vi "SetUpLeCroy.vi"(6 "Therapy (T)":bool, 7 "Therapy VISA session":refnum<visa-resource-name>, 8 "Ann Array Params":T2={"Synth Foc?"=FALSE, "Focal Zones"=41, "Switch T/R"=0, "Trans Geometry (mm)"={"Transducer"=0, "Geo Focus"=12.0, "a (radius)"=3.0, "# of rings"=5, "kerf space "=0.1, "Center Freq"=12.0}, "Sub Ap Excite?"=FALSE, "Full Array Scan?"=FALSE, "Xmt/Rcv"={"XMIT"=[TRUE, TRUE, TRUE, TRUE, TRUE], "RCV"=[TRUE, TRUE, TRUE, TRUE, TRUE]}, "PulseSpacing (us)"=0.0, "Xmit Ring"=0, "XMIT CHS"=0, "RCV CHS"=0, "GPU?"=FALSE, "Save TIFF?"=FALSE, "downfactor"=1, "RCV 1CH"=0} {"RCV 1CH" items=["All", "1", "2", "3", "4", "5"]; "Trans Geometry (mm)"."Transducer" items=["6D 12R 40 MHz"=0, "10D 31R 20 MHz"=1, "10D 23R 20 MHz"=2, "6D 23R 40 MHz"=3, "4.5D 10.7R 40 MHz"=4, "9D 23.5R 20 MHz"=5, "9D 25.8R 20MHz"=6, "Enter"=99]; "Switch T/R" min=1 max=5 step=1}, 10 "Motion Settings In":T6={"No Motion?"=FALSE, "Motion System"=enum."NI 735x", "Motion Bd ID"=1, "Motion Profile"="SMAC1", "# Axis"=1, "Reverse Z axis?"=TRUE, "SMAC Axis"=0, "scan pair"=enum."y-(x) scan", "RT fps"=6.0, "Steps per mm"=[1000, 1000, 1000, 1000], "Motor Parameters"={"velocity ct/s"=[10000.0, 10000.0, 10000.0, 50000.0], "accel ct/s^2"=[50000.0, 50000.0, 50000.0, 200000.0]}, "One Way Scan"=FALSE, "Reverse One Way Scan"=FALSE, "Global Position (mm)"=[], "Plane"=0, "Distance between\nscan lines (um)"=0.0, "Distance between\nscan planes (um)"=0.0, "number of scan planes"=1, "Total steps in line"=0, "Xtra plane\ndistance  (um)"=100, "Xtra planes "=1, "Add Axis"=FALSE, "overshoot cts"=200, "BKPT Shift"=0, "Scan Start Time (ms)"=0, "ESP VISA"="GPIB::1::INSTR", "3rd Axis"=1, "GL Ref Out"=refnum, "Galil Address"=""} {"3rd Axis" items=["x", "y", "z", "w"]; "Xtra planes" min=1; "Xtra plane\ndistance  (um)" min=0; "Distance between\nscan planes (um)" format="%.2f"; "Distance between\nscan lines (um)" format="%.2f"; "SMAC Axis" items=["None"=0, "Axis 1"=1, "Axis 2"=2, "Axis 3"=3, "Axis 4"=4, "Axis 5"=5, "Axis 6"=6, "Axis 7"=7, "Axis 8"=8, "Vector Space 1"=17, "Vector Space 2"=18, "Vector Space 3"=19, "Vector Space 4"=20]; "Motion Bd ID" min=1 max=32 step=1}, 11 "Digitizer Settings":T10={"Digitizer delay (us) "=0.0, "rf points per line"=2048, "lines per plane"=128, "Samp Rate (Hz)"=100000000.0, "Additional dig delay (us)"=0.0, "Voltage Scale"=0.4, "Pre-Looks"=0, "Offset delay (us)"=0.0, "bits A/D"=8, "Avg Num"=1, "DigTimeOut"=5.0, "Rel Dig Delay"=0.0, "Dig Ch"=0, "LeCroyCluster"={"LeCroy Channels"=[TRUE, FALSE, FALSE, FALSE], "LC read pt offset"=0.0, "Sweep Avg"=FALSE}, "Main Digitizer"=enum."NI Digitizer", "Dig Config"=enum."Single channel", "Digitizer ID Cluster"={"Acqiris/Alazar/SP ID"=[], "NI Instr Handles"=[], "LeCroy VISA"="", "GaGe Handle"={"Handle"=0, "Sample size"=0, "Resolution"=0, "Offset"=0, "Channels"=0, "Boards"=0}, "ATS Ref"="ATS9350", "Acqiris Address"=["PCI::INSTR0"], "ADQRef"=refnum, "adq_cu_ptr"=refnum}, "Trigger Settings"={"Trig Source"=1, "Trig Coupling"=0, "Trig Slope"=0, "Level (mV)"=1500.0}, "Bulk Acq"=FALSE, "Bulk Start Indexes"=[], "Data Ref RF"=refnum, "NI ID/Channel"=[], "Total Dig CH"=1, "Xtra Ann Trig delay (us)"=10.0, "Fix Z Delay?"=FALSE, "One Way Transmission?"=FALSE, "Data Ref Log"=refnum} {"Trigger Settings"."Trig Slope" items=["Positive", "Negative"]; "Trigger Settings"."Level (mV)" format="%.2f"; "Trigger Settings"."Trig Coupling" items=["DC 1 MOhm", "AC 1 MOhm", "DC 50 Ohm", "AC 50 Ohm"]; "Trigger Settings"."Trig Source" items=["Chan 1", "External"]; "Rel Dig Delay" format="%.2f"; "DigTimeOut" format="%.2f"; "Avg Num" min=1; "Offset delay (us)" format="%.2f"; "Additional dig delay (us)" format="%.2f"; "Digitizer delay (us)" format="%.2f"}) -> (0 "Waveform Graph":cluster{i32, dbl, dbl[]}(graph), 1 "Equivalent RT delay\ndistance (mm)":dbl=1.5 format="%.4f", 2 "Motion Settings Out":T6={"No Motion?"=FALSE, "Motion System"=enum."NI 735x", "Motion Bd ID"=1, "Motion Profile"="SMAC1", "# Axis"=1, "Reverse Z axis?"=TRUE, "SMAC Axis"=0, "scan pair"=enum."y-(x) scan", "RT fps"=6.0, "Steps per mm"=[1000, 1000, 1000, 1000], "Motor Parameters"={"velocity ct/s"=[10000.0, 10000.0, 10000.0, 50000.0], "accel ct/s^2"=[50000.0, 50000.0, 50000.0, 200000.0]}, "One Way Scan"=FALSE, "Reverse One Way Scan"=FALSE, "Global Position (mm)"=[], "Plane"=0, "Distance between\nscan lines (um)"=0.0, "Distance between\nscan planes (um)"=0.0, "number of scan planes"=1, "Total steps in line"=0, "Xtra plane\ndistance  (um)"=100, "Xtra planes "=1, "Add Axis"=FALSE, "overshoot cts"=200, "BKPT Shift"=0, "Scan Start Time (ms)"=0, "ESP VISA"="GPIB::1::INSTR", "3rd Axis"=1, "GL Ref Out"=refnum, "Galil Address"=""} {"3rd Axis" items=["x", "y", "z", "w"]; "Xtra planes" min=1; "Xtra plane\ndistance  (um)" min=0; "Distance between\nscan planes (um)" format="%.2f"; "Distance between\nscan lines (um)" format="%.2f"; "SMAC Axis" items=["None"=0, "Axis 1"=1, "Axis 2"=2, "Axis 3"=3, "Axis 4"=4, "Axis 5"=5, "Axis 6"=6, "Axis 7"=7, "Axis 8"=8, "Vector Space 1"=17, "Vector Space 2"=18, "Vector Space 3"=19, "Vector Space 4"=20]; "Motion Bd ID" min=1 max=32 step=1}, 3 "Ann Array Params out":T2={"Synth Foc?"=FALSE, "Focal Zones"=41, "Switch T/R"=0, "Trans Geometry (mm)"={"Transducer"=0, "Geo Focus"=12.0, "a (radius)"=3.0, "# of rings"=5, "kerf space "=0.1, "Center Freq"=12.0}, "Sub Ap Excite?"=FALSE, "Full Array Scan?"=FALSE, "Xmt/Rcv"={"XMIT"=[TRUE, TRUE, TRUE, TRUE, TRUE], "RCV"=[TRUE, TRUE, TRUE, TRUE, TRUE]}, "PulseSpacing (us)"=0.0, "Xmit Ring"=0, "XMIT CHS"=0, "RCV CHS"=0, "GPU?"=FALSE, "Save TIFF?"=FALSE, "downfactor"=1, "RCV 1CH"=0} {"RCV 1CH" items=["All", "1", "2", "3", "4", "5"]; "Trans Geometry (mm)"."Transducer" items=["6D 12R 40 MHz"=0, "10D 31R 20 MHz"=1, "10D 23R 20 MHz"=2, "6D 23R 40 MHz"=3, "4.5D 10.7R 40 MHz"=4, "9D 23.5R 20 MHz"=5, "9D 25.8R 20MHz"=6, "Enter"=99]; "Switch T/R" min=1 max=5 step=1}, 4 "Digitizer Settings Out":T10={"Digitizer delay (us) "=0.0, "rf points per line"=2048, "lines per plane"=128, "Samp Rate (Hz)"=100000000.0, "Additional dig delay (us)"=0.0, "Voltage Scale"=0.4, "Pre-Looks"=0, "Offset delay (us)"=0.0, "bits A/D"=8, "Avg Num"=1, "DigTimeOut"=5.0, "Rel Dig Delay"=0.0, "Dig Ch"=0, "LeCroyCluster"={"LeCroy Channels"=[TRUE, FALSE, FALSE, FALSE], "LC read pt offset"=0.0, "Sweep Avg"=FALSE}, "Main Digitizer"=enum."NI Digitizer", "Dig Config"=enum."Single channel", "Digitizer ID Cluster"={"Acqiris/Alazar/SP ID"=[], "NI Instr Handles"=[], "LeCroy VISA"="", "GaGe Handle"={"Handle"=0, "Sample size"=0, "Resolution"=0, "Offset"=0, "Channels"=0, "Boards"=0}, "ATS Ref"="ATS9350", "Acqiris Address"=["PCI::INSTR0"], "ADQRef"=refnum, "adq_cu_ptr"=refnum}, "Trigger Settings"={"Trig Source"=1, "Trig Coupling"=0, "Trig Slope"=0, "Level (mV)"=1500.0}, "Bulk Acq"=FALSE, "Bulk Start Indexes"=[], "Data Ref RF"=refnum, "NI ID/Channel"=[], "Total Dig CH"=1, "Xtra Ann Trig delay (us)"=10.0, "Fix Z Delay?"=FALSE, "One Way Transmission?"=FALSE, "Data Ref Log"=refnum} {"Trigger Settings"."Trig Slope" items=["Positive", "Negative"]; "Trigger Settings"."Level (mV)" format="%.2f"; "Trigger Settings"."Trig Coupling" items=["DC 1 MOhm", "AC 1 MOhm", "DC 50 Ohm", "AC 50 Ohm"]; "Trigger Settings"."Trig Source" items=["Chan 1", "External"]; "Rel Dig Delay" format="%.2f"; "DigTimeOut" format="%.2f"; "Avg Num" min=1; "Offset delay (us)" format="%.2f"; "Additional dig delay (us)" format="%.2f"; "Digitizer delay (us)" format="%.2f"})   [LabVIEW 2022 SP3]
uses:
  -DigitizerRoutines/DigitizerSettings.ctl
  -DigitizerRoutines/Digitizer.ctl
  -DigitizerRoutines/DigConfig.ctl
  -DigitizerRoutines/DigitizerID.ctl
  C:/Windows/System32/ADQAPI_dotNet_helper.dll
  Motion Controllers/NI_controller/-NI_MotionRoutines/MotionParameters.ctl
  Motion Controllers/NI_controller/-NI_MotionRoutines/MotionSys.ctl
  Motion Controllers/-MotionRoutines/ScanAxis.ctl
  Motion Controllers/-MotionRoutines/3rdAxis.ctl
  Annular Array/-AnnularRoutines/AnnularArray.ctl
  Annular Array/-AnnularRoutines/TransGeometry.ctl
  Annular Array/-AnnularRoutines/ArrayGeometry.ctl
  Motion Controllers/Galil/Command Menu.ctl
  <vilib>/Analysis/baseanly.llb/Mean (DBL).vi
  Motion Controllers/-MotionRoutines/MotionGlobals.vi
  Pulsers/PulserGlobals.vi
  Switch Modules/SwitchGlobals.vi
  <instrlib>/LeCroy Wave Series/Public/Configure/Configure Edge Trigger.vi
  <vilib>/Utility/file.llb/Write Delimited Spreadsheet (DBL).vi
  <vilib>/Analysis/NI_AALPro.lvlib
  <instrlib>/LeCroy Wave Series/LeCroy Wave Series.lvlib
  <vilib>/Analysis/NI_AALBase.lvlib
  <vilib>/Motion/FlexMotion/FunctionsVIs/StartStopMotion.llb/Start Motion (8 axes).flx
  <vilib>/Motion/FlexMotion/FunctionsVIs/StartStopMotion.llb/Stop Motion (8 axes).flx
panel:
  in  "Filter Prameters":T1={"low cutoff"=5, "order"=81, "high cutoff"=65}
  in  "T/R Channel":u32(slide)=1 min=1 max=8 step=1 scale=1.0..5.0
  in  "prf (kHz)":dbl=1.0 format="%.3f"
  in  "rf points per line":i32=2048 min=1
  in  "Delay (us)":dbl format="%.2f"
  out "Sample Rate":sgl(ring) items=["40 GS/s"=40000, "20 GS/s"=20000, "10 GS/s"=10000, "5 GS/s"=5000, "2.5 GS/s"=2500, "1.25 GS/s"=1250, "500 MS/s"=500, "250 MS/s"=250, "100 MS/s"=100, "50 MS/s"=50, "25 MS/s"=25, "10 MS/s"=10, "5 MS/s"=5, "2.5 MS/s"=2.5, "1 MS/s"=1, "500 kS/s"=0.5, "250 kS/s"=0.25, "100 kS/s"=0.1, "50 kS/s"=0.05, "25 kS/s"=0.025, "10 kS/s"=0.01, "5 kS/s"=0.005, "2.5 kS/s"=0.0025, "1 kS/s"=0.001]
  out "Total Delay (us)":dbl=1.5 format="%.3f"
  in  "Channel tab":enum32{"C1", "C2", "C3", "C4"}(tab)
  in  "Voltage/DIV CH1":sgl=2.0
  in  "Voltage/DIV CH2":sgl=2.0
  in  "Voltage/DIV CH3":sgl=2.0
  in  "Voltage/DIV CH4":sgl=2.0
  in  "Time/Div":dbl(ring)=5.0 items=["5 ks"=5000.0, "2 ks"=2000.0, "1 ks"=1000.0, " 500 s"=500.0, " 200 s"=200.0, "100 s"=100.0, " 50 s"=50.0, "20 s"=20.0, "10 s"=10.0, "5 s"=5.0, "2 s"=2.0, "1 s"=1.0, "500 ms"=0.5, "200 ms"=0.2, " 100 ms"=0.1, "50 ms"=0.05, "20 ms"=0.02, "10 ms"=0.01, "5 ms"=0.005, "2 ms"=0.002, "1 ms"=0.001, "500 us"=0.0005, "200 us"=0.0002, "100 us"=0.0001, "50 us"=5e-05, "20 us"=2e-05, "10 us"=1e-05, "5 us"=5e-06, "2 us"=2e-06, "1 us"=1e-06, "500 ns"=5e-07, "200 ns"=2e-07, "100 ns"=1e-07, "50 ns"=5e-08, "20 ns"=2e-08, "10 ns"=1e-08, "5 ns"=5e-09, "2 ns"=2e-09, "1 ns"=1e-09, "500 ps"=5e-10, "200 ps"=2e-10, "100 ps"=1e-10, "50 ps"=5e-11, "20 ps"=2e-11]
  in  "Lecroy Setup":T5(ring)
  in  "Load Lecroy Setup":bool
  in  "Inc Step\nSize (mm)":dbl=0.5
  in  "Stop Motor":bool
  in  "Axis":enum32{"Axis 1", "Axis 2", "Axis 3", "Axis 4"}(radio)
  in  "Position (mm) (Abs)":dbl format="%.3f"
  in  "offset delay":dbl
  out "read pt offset":dbl
  in  "Delay Corr?":bool=TRUE
  in  "Gate duration (mics)":dbl=12.0 min=0.025
  in  "Func Gen":u16(ring)=1 items=["Agilent", "Tabor"]
  in  "Custom Waveform":bool
  in  "Man Cont":bool
  in  "Save trace?":bool
  out "Lines in burst":i32=1 min=1 max=50000 step=1
  in  "cycles (f), time(t)":bool=TRUE
  in  "Set Pulser":bool
  in  "go to scan type":bool
  in  "Therapy Burst Set Up":T14={"Therapy Set Up"={"Cycles"=1.0, "Frequency (MHz)"=40.0, "Amplitude (mV)"=200.0}, "Divide prf by"=1, "Therapy Delay (ms) "=10.0, "Counter On (T)"=TRUE} {"Therapy Delay (ms)" min=0.025 format="%.3f"; "Therapy Set Up"."Amplitude (mV)" min=50.0 max=1000.0 format="%.2f"; "Therapy Set Up"."Frequency (MHz)" min=0.01 max=200.0 format="%.4f"; "Therapy Set Up"."Cycles" min=1 max=50000 step=1 format="%.3f"}
  in  "ExitSendCmd":bool
  # "Digitizer Settings"
  # "Voltage Scales"
  # "Position Adjustment"
  # "Yellow curser used for additional delay. RF data is captured between yellow and red lines."
  # "Key Board Short Cuts\nX: \t      Autoscale in X\nY: \t      Autoscale in Y\nSpace Bar:           Exit\nShift:           Step * 0.1\nCtrl:          Step * 0.01"
  # "Z: \t\t             +W\nC: \t\t              -W\nPageUp:      \t+Z\nPageDown:\t   -Z\nUp Arrow:\t    +Y\nDown Arrow: \t-Y\nLeft Arrow: \t  +X\nRight Arrow:  -X"
  # "© 2000-2022 WCM"
  # "1-D and 2-D B scan settings"
  # "1-D and 2-D B scan settings"
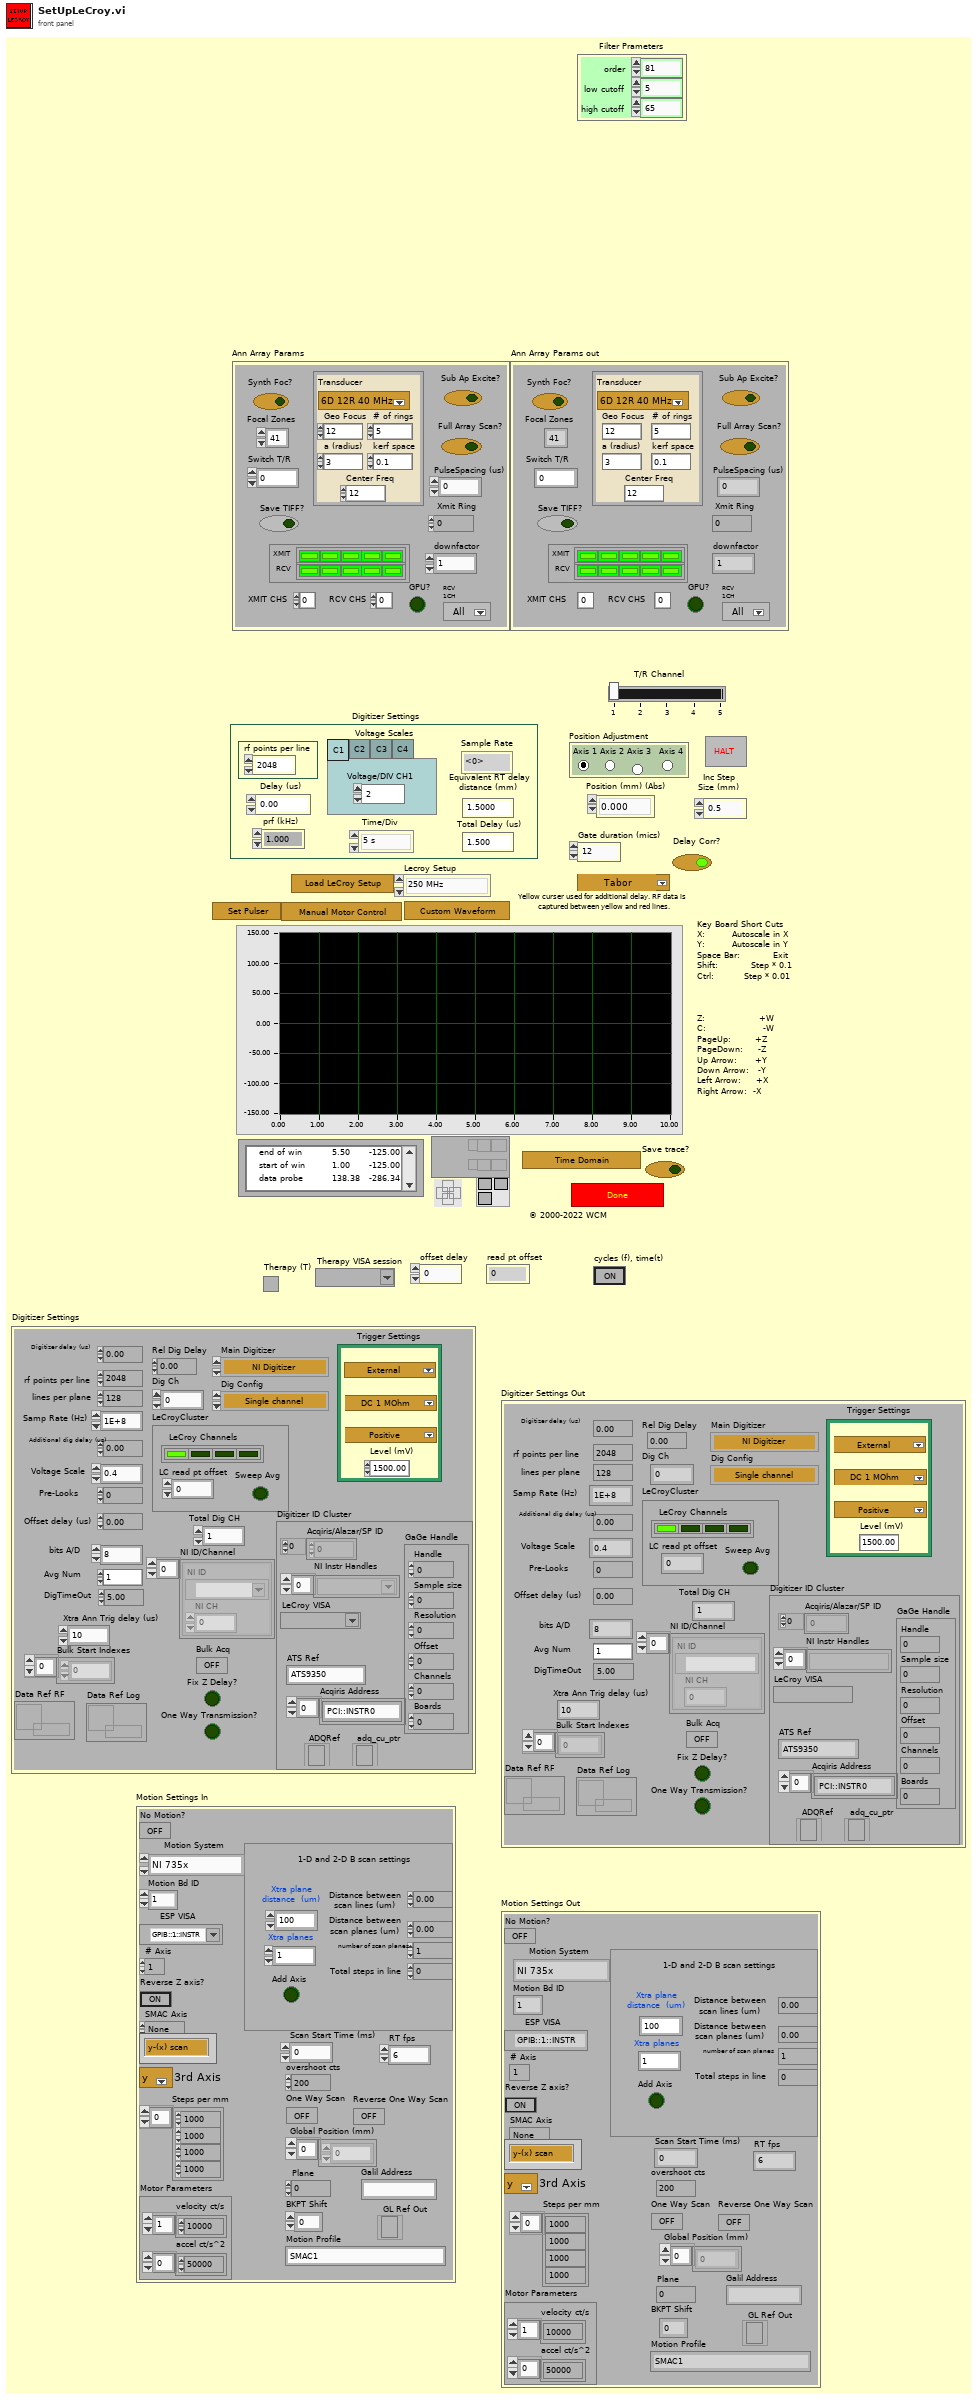
[diagram p1: front panel]
types:
  T1 = cluster{"low cutoff":i32, "order":i32, "high cutoff":i32}
  T2 = typedef "AnnularArray.ctl" = cluster{"Synth Foc?":bool, "Focal Zones":i16, "Switch T/R":i16, "Trans Geometry (mm)":T3, "Sub Ap Excite?":bool, "Full Array Scan?":bool, "Xmt/Rcv":cluster{"XMIT":bool[], "RCV":bool[]}, "PulseSpacing (us)":sgl, "Xmit Ring":i32, "XMIT CHS":u8, "RCV CHS":u8, "GPU?":bool, "Save TIFF?":bool, "downfactor":i32, "RCV 1CH":u16}
  T3 = typedef "TransGeometry.ctl" = cluster{"Transducer":T4, "Geo Focus":dbl, "a (radius)":dbl, "# of rings":i32, "kerf space ":dbl, "Center Freq":dbl}
  T4 = typedef "ArrayGeometry.ctl" = u16
  T5 = enum16{"250 MHz", "250 MHz Focus", "Opti 250", "500 MHz", "500 MHz Focus", "500 MHz New"}
  T6 = typedef "MotionParameters.ctl" = cluster{"No Motion?":bool, "Motion System":T7, "Motion Bd ID":u8, "Motion Profile":string, "# Axis":i8, "Reverse Z axis?":bool, "SMAC Axis":u16, "scan pair":T8, "RT fps":sgl, "Steps per mm":i32[], "Motor Parameters":cluster{"velocity ct/s":dbl[], "accel ct/s^2":dbl[]}, "One Way Scan":bool, "Reverse One Way Scan":bool, "Global Position (mm)":dbl[], "Plane":i32, "Distance between\nscan lines (um)":sgl, "Distance between\nscan planes (um)":sgl, "number of scan planes":i32, "Total steps in line":i32, "Xtra plane\ndistance  (um)":i32, "Xtra planes ":i32, "Add Axis":bool, "overshoot cts":i32, "BKPT Shift":i32, "Scan Start Time (ms)":u32, "ESP VISA":refnum<visa-resource-name>, "3rd Axis":T9, "GL Ref Out":refnum<k7>, "Galil Address":string}
  T7 = typedef "MotionSys.ctl" = enum16{"MM3000", "NI 735x", "Newport ESP", "No Motion Card", "Galil"}
  T8 = typedef "ScanAxis.ctl" = enum16{"y-(x) scan", "x-(y) scan", "z-(x) scan", "z-(y) scan", "y-(z) scan", "x-(z) scan", "w-(x) scan", "w-(y) scan", "w-(z) scan", "x-(w) scan", "y-(w) scan", "z-(w) scan"}
  T9 = typedef "3rdAxis.ctl" = u16
  T10 = typedef "DigitizerSettings.ctl" = cluster{"Digitizer delay (us) ":dbl, "rf points per line":i32, "lines per plane":i32, "Samp Rate (Hz)":dbl, "Additional dig delay (us)":dbl, "Voltage Scale":dbl, "Pre-Looks":i32, "Offset delay (us)":dbl, "bits A/D":i8, "Avg Num":i32, "DigTimeOut":sgl, "Rel Dig Delay":sgl, "Dig Ch":i32, "LeCroyCluster":cluster{"LeCroy Channels":bool[], "LC read pt offset":dbl, "Sweep Avg":bool}, "Main Digitizer":T11, "Dig Config":T12, "Digitizer ID Cluster":T13, "Trigger Settings":cluster{"Trig Source":u16, "Trig Coupling":u16, "Trig Slope":u16, "Level (mV)":dbl}, "Bulk Acq":bool, "Bulk Start Indexes":i32[], "Data Ref RF":refnum<data-value>, "NI ID/Channel":cluster{"NI ID":refnum<k15>, "NI CH":i32}[], "Total Dig CH":i32, "Xtra Ann Trig delay (us)":dbl, "Fix Z Delay?":bool, "One Way Transmission?":bool, "Data Ref Log":refnum<data-value>}
  T11 = typedef "Digitizer.ctl" = enum16{"Acqiris Digitizer", "NI Digitizer", "LeCroy", "GaGe", "AlazarTech", "No Digitizer", "Teledyne"}
  T12 = typedef "DigConfig.ctl" = enum16{"Single channel", "2 Chans w/ 2 Acqiris", "2 Chans w/ 1 Acqiris", "5-CH Pulser New", "5-CH pulser w/ ann array", "5-pass style ann array", "Empty"}
  T13 = typedef "DigitizerID.ctl" = cluster{"Acqiris/Alazar/SP ID":u32[], "NI Instr Handles":refnum<k15>[], "LeCroy VISA":refnum<visa-resource-name>, "GaGe Handle":cluster{"Handle":u32, "Sample size":u32, "Resolution":i32, "Offset":i32, "Channels":u32, "Boards":u32}, "ATS Ref":string, "Acqiris Address":string[], "ADQRef":refnum<k24>, "adq_cu_ptr":refnum<k24>}
  T14 = cluster{"Therapy Set Up":cluster{"Cycles":sgl, "Frequency (MHz)":dbl, "Amplitude (mV)":dbl}, "Divide prf by":i32, "Therapy Delay (ms) ":dbl, "Counter On (T)":bool}
  T15 = typedef "EKG_Mode.ctl" = u16
  T16 = typedef "location.ctl" = enum16{"Automatic", "WCM Main", "Hawaii", "Columbia MM3000", "Columbia  NI System", "NYU", "RRI 2", "UHI Allen", "CUMC RT", "Chiba", "Stony Brook", "WCM Microscopy", "WCM Aeoretch", "WCM Optics Lab", "WCM Main 2Axis", "WCM Rotation", "WCM SAM SMAC", "SERI GP"}
  T17 = typedef "SwitchOption.ctl" = enum16{"Cytex", "Pickering", "NI Switch", "No Switch", "Riverside USB"}
  T18 = typedef "Command Menu.ctl" = enum16{"CommandPassThrough", "Abort Motion", "Define Pos", "Velocity", "Acceleration", "Deceleration", "Position Rel", "Postion Abs", "Begin Move", "After Move", "Home", "KI", "KD", "KP", "IL", "Config I/O", "Set Bit", "Clear Bit", "Motor Off", "Moto On", "Status", "Execute", "Halt Execute", "HX Status", "Tell Velocity", "Check Motion", "BreakPoint", "Tell Position", "Current Code Line", "Tell Switches", "OC Force On", "OC Off", "Pos Soft Limit", "Rev Soft Limit"}
  T19 = cluster{"Therapy frequency (MHz)":dbl, "Therapy amplitude (mV)":dbl, "time therapy on (s)":dbl, "Therapy Delay (ms) ":dbl, "Time (s)":dbl}
  T20 = cluster{"time therapy on (s)":dbl, "Therapy frequency (MHz)":dbl, "Therapy amplitude (mV)":dbl}
  T21 = typedef "pulser.ctl" = enum16{"Pan 5900", "Daxsonics", "Agilent 33xxx", "UTEX", "JSR", "WMC Mono-Cycle", "No Pulser", "NYU AVTECH", "Tabor W1281A", "Pan 5800", "Unlisted", "Tabor WX2182B"}
  T22 = typedef "eventvkey.ctl" = enum16{"ASCII", "Enter", "Return", "Shift", "Ctrl", "Alt", "Cmd", "Opt", "Caps", "NumLock", "Clear", "Break", "Up", "Down", "Left", "Right", "Insert", "Delete", "Home", "End", "PageUp", "PageDown", "Escape", "Help", "Pause", "ScrollLock", "F1", "F2", "F3", "F4", "F5", "F6", "F7", "F8", "F9", "F10", "F11", "F12", "F13", "F14", "F15", "F16", "F17", "F18", "F19", "F20", "F21", "F22", "F23", "F24", "Play", "VolumeUp", "VolumeDown", "Mute", "Two Byte Char"}
  T23 = cluster{"Shift":bool, "Ctrl":bool, "Alt":bool, "Cmd":bool, "Opt":bool}
  T24 = cluster{"Cycles":sgl, "Frequency (MHz)":dbl, "Amplitude (mV)":dbl}
  T25 = typedef "Resource Out (Enum).flx" = u16
  T26 = typedef "Bd Id Out" = u8
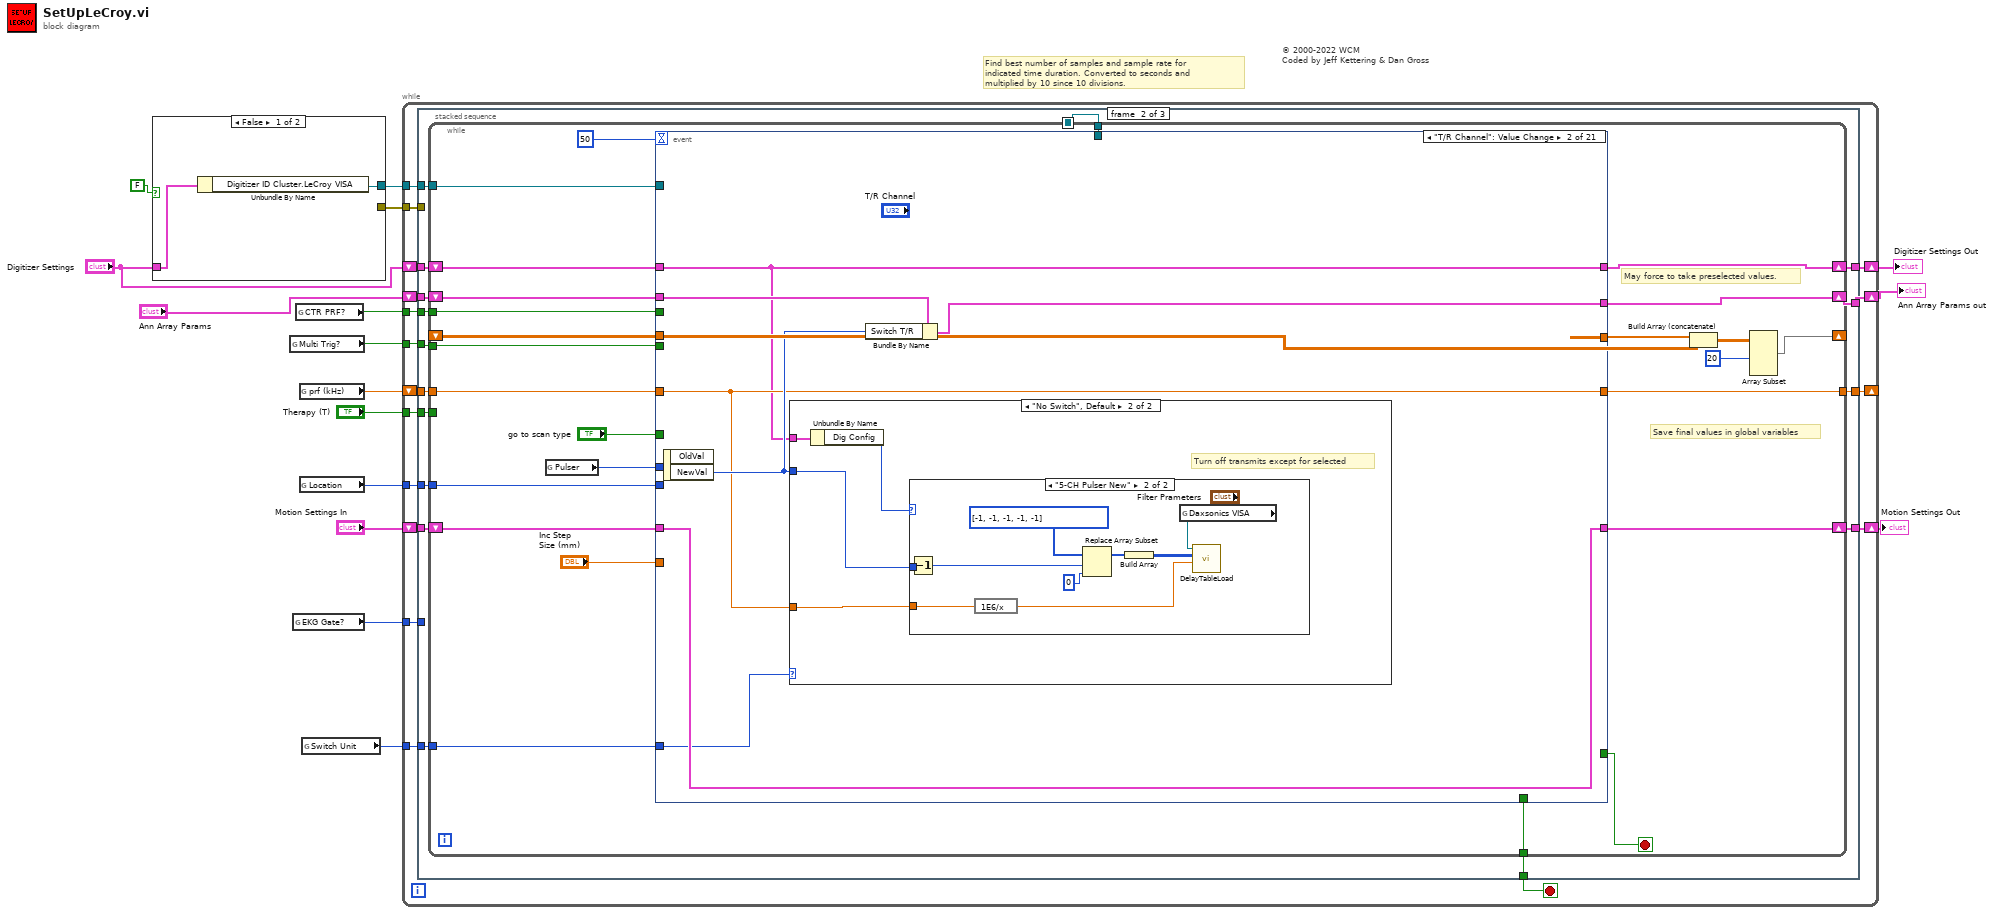
[diagram p0: block diagram]
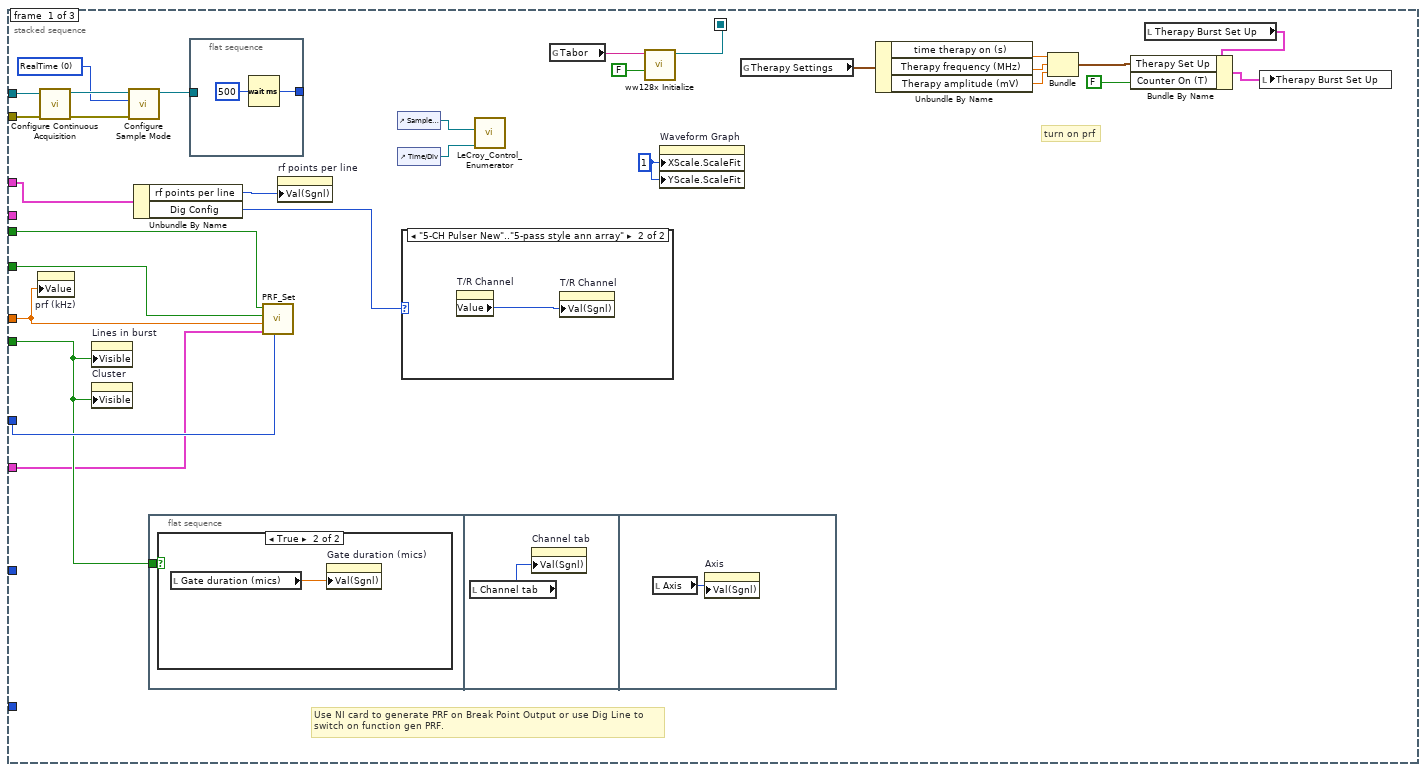
[diagram p2: hidden frame]
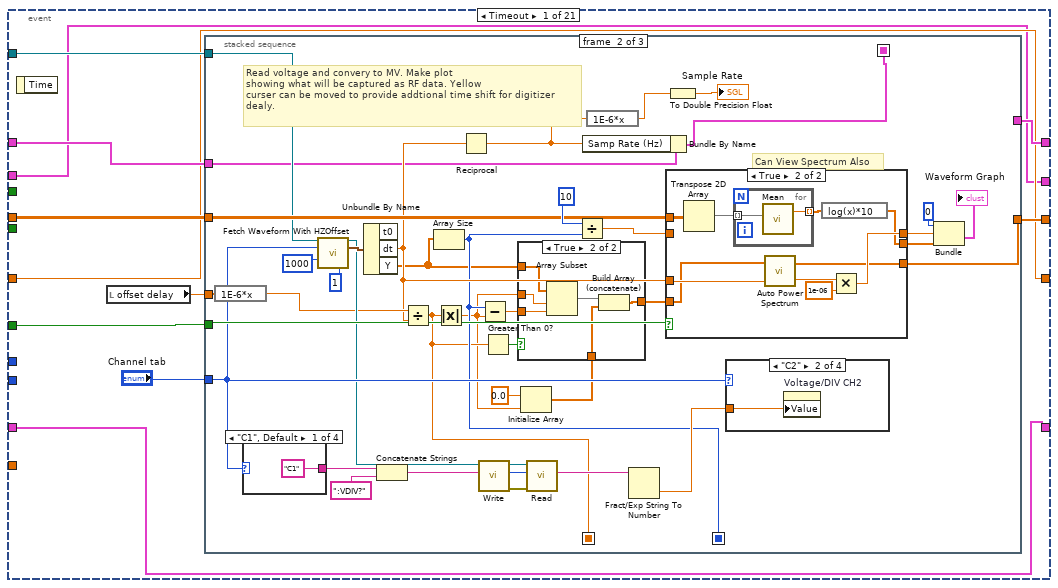
[diagram p5: hidden frame]
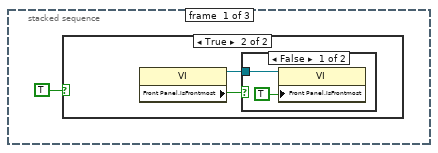
[diagram p6: hidden frame]
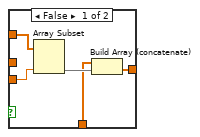
[diagram p9: hidden frame]
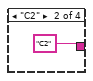
[diagram p10: hidden frame]
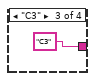
[diagram p11: hidden frame]
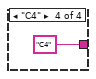
[diagram p12: hidden frame]
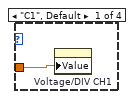
[diagram p13: hidden frame]
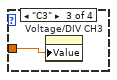
[diagram p14: hidden frame]
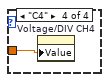
[diagram p15: hidden frame]
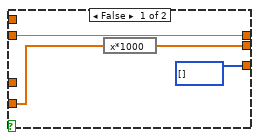
[diagram p16: hidden frame]
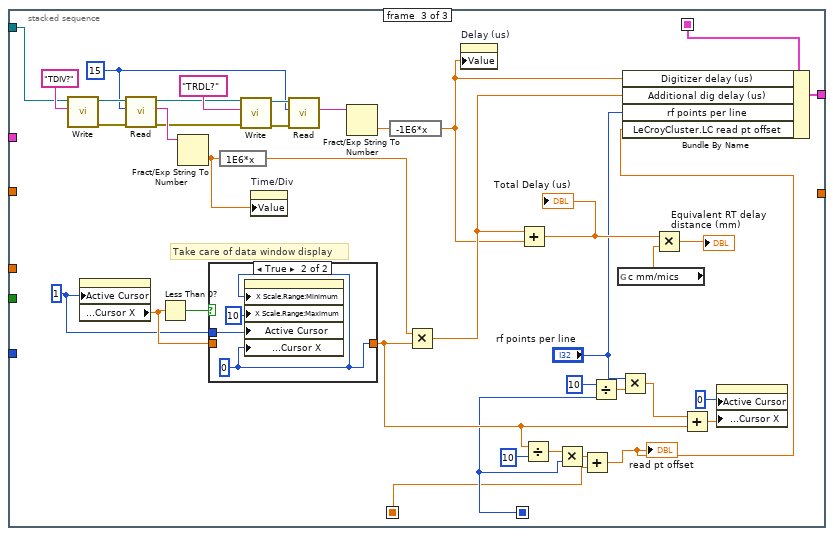
[diagram p17: hidden frame]
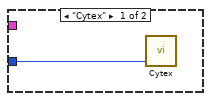
[diagram p19: hidden frame]
diagram:
  # "Find best number of samples and sample rate for indicated time duration. Converted to seconds and multiplied by 10 since 10 divisions."
  # "© 2000-2022 WCM\nCoded by Jeff Kettering & Dan Gross"
  n1 = case shown="False" FALSE {
    tunnel: [w17 w21] -> w13
    tunnel: [_ w19] -> w12
    tunnel: "Digitizer Settings" -> [w18 _]
    frame False {
      n2 = Unbundle By Name(w18) -> ("Digitizer ID Cluster.LeCroy VISA"=w17:refnum<visa-resource-name>)
    }
    frame True {
      n3 = call <instrlib>:"Initialize.vi"("Reset? (T: Yes)"=FALSE, "VISA resource name"=refnum<visa-resource-name> "VICP::LCRY0604P14300") -> ("error out"=w19:errorcluster, "VISA resource name out"=w21:refnum<visa-resource-name>)  [unwired: 2 in, 6 out]
    }
  }
  n4 = global read "MotionGlobals.vi" "Multi Trig?"() -> (w9:bool)
  n5 = global read "MotionGlobals.vi" "EKG Gate?"() -> (w14:T15)
  n6 = global read "MotionGlobals.vi" "CTR PRF?"() -> (w10:bool)
  n7 = global read "PulserGlobals.vi" "prf (kHz)"() -> (w4:dbl)
  n8 = global read "MotionGlobals.vi" "Location"() -> (w15:T16)
  n9 = global read "SwitchGlobals.vi" "Switch Unit"() -> (w1:T17)
  n10 = while {
    tunnel: "Therapy (T)" -> [w39]
    tunnel: w15 -> [w38]
    tunnel: w14 -> [w37]
    tunnel: w13 -> [w36]
    tunnel: w12 -> [w35]
    tunnel: w10 -> [w34]
    tunnel: w9 -> [w33]
    shift-right: [w32] -> w8
    shift-left: "Digitizer Settings" -> [w31]
    shift-right: [w30] -> w6
    shift-left: "Motion Settings In" -> [w29]
    shift-right: [w27] -> _
    shift-left: w4 -> [w28]
    shift-right: [w24] -> w2
    shift-left: "Ann Array Params" -> [w25]
    tunnel: w1 -> [w23]
    stop <- w26 stop-if-true
    n11 = stacked-sequence {
      seq-local: [w64 _ _] -> [_ w90 w568]
      tunnel: w39 -> [w62 w91 w572]
      tunnel: w38 -> [w66 w81 w575]
      tunnel: w36 -> [w60 w89 _]
      tunnel: w37 -> [_ _ w574]
      tunnel: w28 -> [w45 w88 _]
      tunnel: w35 -> [w59 _ _]
      tunnel: w34 -> [w55 w83 w570]
      tunnel: w33 -> [w54 w82 w569]
      tunnel: w31 -> [w47 w87 _]
      tunnel: [_ w86 _] -> w32
      tunnel: w29 -> [w44 w85 w567]
      tunnel: [_ w84 _] -> w30
      tunnel: [_ w80 _] -> w27
      tunnel: [_ w79 _] -> w26
      tunnel: w25 -> [_ w78 _]
      tunnel: [_ w77 _] -> w24
      tunnel: w23 -> [_ w76 _]
      frame #0 {
        w41 = u8 1 ("X Scale.Scale Fit")
        w56 = u16 0 items=["RealTime", "RIS", "Sequence", "Roll", "WaveStream"] ("Sample Mode (0: RealTime)")
        # "turn on prf"
        # "Use NI card to generate PRF on Break Point Output or use Dig Line to switch on function gen PRF."
        n12 = property on="prf (kHz)" class="DigNum (strict)"("Value"=w45) -> ()  [unwired: 2 in, 2 out]
        n13 = call <instrlib>:"Configure Continuous Acquisition.vi"("error in (no error)"=w59, "VISA resource name"=w60) -> ("error out"=w58:errorcluster, "VISA resource name out"=w57:refnum<visa-resource-name>)  [unwired: 8 in]
        n14 = property on="Lines in burst" class="DigNum (strict)"("Visible"=w62) -> ()  [unwired: 2 in, 2 out]
        n15 = property on="Cluster" class="Clust (strict)"("Visible"=w62) -> ()  [unwired: 2 in, 2 out]
        n16 = call <instrlib>:"Configure Sample Mode.vi"("error in (no error)"=w58, "Sample Mode (0: RealTime)"=w56, "VISA resource name"=w57) -> ("VISA resource name out"=w53:refnum<visa-resource-name>)  [unwired: 7 in, 1 out]
        n17 = Unbundle By Name(w47) -> ("rf points per line"=w46:i32, "Dig Config"=w40:T12)
        n18 = flat-sequence {
          tunnel: w62 -> [w72]
          frame #0 {
            n19 = case shown="True" w72 {
              frame False {
              }
              frame True {
                n20 = local read "Gate duration (mics)"() -> (w73:dbl)
                n21 = property on="Gate duration (mics)" class="DigNum (strict)"("Val(Sgnl)"=w73) -> ()  [unwired: 2 in, 2 out]
              }
            }
          }
          frame #1 {
            n22 = local read "Channel tab"() -> (w74:enum32{"C1", "C2", "C3", "C4"})
            n23 = property on="Channel tab" class="TabCtl (strict)"("Val(Sgnl)"=w74) -> ()  [unwired: 2 in, 2 out]
          }
          frame #2 {
            n24 = local read "Axis"() -> (w75:enum32{"Axis 1", "Axis 2", "Axis 3", "Axis 4"})
            n25 = property on="Axis" class="RadioBtnsControl (strict)"("Val(Sgnl)"=w75) -> ()  [unwired: 2 in, 2 out]
          }
        }
        n26 = flat-sequence {
          tunnel: w53 -> [_]
          tunnel: [w70] -> _
          frame #0 {
            n27 = Wait (ms)(milliseconds to wait=u32 500) -> (millisecond timer value=w70:u32)
          }
        }
        n28 = call "PRF_Set.vi"("Location"=w66, "Motion Settings In"=w44, "prf (kHz)"=w45, "Multi Trig?"=w54, "CTR PRF?"=w55) -> ()  [unwired: 7 in]
        n29 = property on="rf points per line" class="DigNum (strict)"("Val(Sgnl)"=w46) -> ()  [unwired: 2 in, 2 out]
        n30 = control-ref of="Sample Rate"() -> (w42:refnum<vi>)
        n31 = control-ref of="Time/Div"() -> (w43:refnum<vi>)
        n32 = case shown="\"5-CH Pulser New\"..\"5-pass style ann array\"" w40 {
          frame "Single channel", Default {
          }
          frame "5-CH Pulser New".."5-pass style ann array" {
            n33 = property on="T/R Channel" class="Slide (strict)"() -> ("Value"=w69:u32)  [unwired: 2 in, 2 out]
            n34 = property on="T/R Channel" class="Slide (strict)"("Val(Sgnl)"=w69) -> ()  [unwired: 2 in, 2 out]
          }
        }
        n35 = call "LeCroy_Control_Enumerator.vi"("Time/Div (S) Ref"=w43, "Sampling Rate (MHz) Ref"=w42) -> ()  [unwired: 7 in, 3 out]
        n36 = global read "PulserGlobals.vi" "Tabor"() -> (w48:string)
        n37 = call <instrlib>:"ww128x Initialize.vi"("reset device (Yes)"=FALSE ("reset device"), "resource name"=w48) -> ("instrument handle out"=w64:refnum<k15>)  [unwired: 2 in, 7 out]
        n38 = property on="Waveform Graph" class="WFGraph (strict)"("XScale.ScaleFit"=w41, "YScale.ScaleFit"=w41) -> ()  [unwired: 2 in, 2 out]
        n39 = global read "PulserGlobals.vi" "Therapy Settings"() -> (w52:T19)
        n40 = Unbundle By Name(w52) -> ("time therapy on (s)"=w50:dbl, "Therapy frequency (MHz)"=w51:dbl, "Therapy amplitude (mV)"=w49:dbl)
        n41 = Bundle("time therapy on (s)"=w50, "Therapy frequency (MHz)"=w51, "Therapy amplitude (mV)"=w49) -> (w61:T20)  [unwired: 1 in]
        n42 = local read "Therapy Burst Set Up"() -> (w63:T14)
        n43 = Bundle By Name(cluster=w63, "Therapy Set Up"=w61, "Counter On (T)"=FALSE) -> (w68:T14)
        n44 = local write "Therapy Burst Set Up"(w68) -> ()
      }
      frame #1 {
        n45 = while {
          shift-left: _ -> [w109]
          shift-right: [w114] -> _
          tunnel: w91 -> [_]
          tunnel: w90 -> [w111]
          tunnel: w89 -> [w108]
          tunnel: w88 -> [w107]
          shift-right: [w104] -> w86
          shift-left: w87 -> [w105]
          shift-right: [w102] -> w84
          shift-left: w85 -> [w103]
          tunnel: w83 -> [w99]
          tunnel: w82 -> [w98]
          tunnel: w81 -> [w97]
          tunnel: [w96] -> w80
          tunnel: [w95] -> w79
          shift-right: [w93] -> w77
          shift-left: w78 -> [w94]
          tunnel: w76 -> [w92]
          stop <- w106 stop-if-true
          # "May force to take preselected values."
          # "Save final values in global variables"
          n46 = global read "PulserGlobals.vi" "Pulser"() -> (w100:T21)
          n47 = event shown="[1] \"T/R Channel\": Value Change" {
            selector: _ -> [_ _ _ _ _ _ _ _ _ _ _ _ _ _ _ _ _ _ _ _ _]
            dyn-events: _ -> [_ _ _ _ _ _ _ _ _ _ _ _ _ _ _ _ _ _ _ _ _]
            timeout: 50 -> [_ _ _ _ _ _ _ _ _ _ _ _ _ _ _ _ _ _ _ _ _]
            tunnel: "go to scan type" -> [w125 _ _ _ _ _ _ _ _ _ _ _ _ w427 _ _ _ _ _ _ _]
            tunnel: w100 -> [_ _ _ _ _ _ w324 w329 _ _ _ _ _ _ _ _ _ _ _ _ _]
            tunnel: w111 -> [_ _ _ _ _ _ _ w331 _ _ _ _ _ _ _ w460 _ _ _ _ _]
            tunnel: w109 -> [w127 _ _ _ _ _ _ _ _ _ _ _ _ _ _ _ _ _ _ _ _]
            tunnel: [w126 _ _ _ _ _ _ _ _ _ _ _ _ _ _ _ _ _ _ _ _] -> w116
            tunnel: w108 -> [w124 _ _ w282 w295 w313 _ _ w336 _ _ _ _ _ _ _ _ _ _ _ _]
            tunnel: w107 -> [w119 w252 w273 w283 w300 w316 w325 w328 w350 w372 w376 w413 _ w421 w441 w453 w468 w477 w503 w532 w556]
            tunnel: [_ _ _ _ _ _ _ _ _ _ _ w405 TRUE _ _ _ _ w476 _ _ _] -> w106
            tunnel: w105 -> [w122 w250 w275 w285 w302 w310 w322 w333 w352 w374 w380 w414 w419 w424 w440 w456 w470 w480 w504 w534 w560]
            tunnel: [w121 w250 w275 w285 w302 w310 w320 w333 w352 w374 w380 w414 w419 w424 w440 w456 w470 w480 w504 w534 w560] -> w104
            tunnel: w103 -> [w120 w255 w274 w284 w301 w317 w326 w332 w351 w373 w379 w396 w418 w423 w439 w454 w469 w479 w492 w530 w559]
            tunnel: [w120 w255 w274 w284 w301 w317 w326 w332 w351 w373 w377 w396 w418 w423 w439 w454 w469 w479 w492 w533 w557] -> w102
            tunnel: "Inc Step\nSize (mm)" -> [_ _ _ _ _ _ _ _ _ _ _ w406 _ _ _ _ _ _ _ _ _]
            tunnel: w99 -> [_ _ _ _ _ _ _ _ _ _ _ _ _ _ _ _ _ _ _ _ _]
            tunnel: w98 -> [_ _ _ _ _ _ _ _ _ _ _ _ _ _ _ _ _ _ _ _ _]
            tunnel: w97 -> [_ _ _ _ _ _ _ _ _ _ _ _ _ _ _ _ _ _ _ _ _]
            tunnel: [w119 w252 w273 w283 w300 w316 w325 w328 w350 w372 w376 w413 "prf (kHz)" w421 w441 w453 w468 w477 w503 w532 w556] -> w96
            tunnel: [_ _ _ _ _ _ _ _ _ _ _ w405 _ _ _ _ _ w476 _ _ _] -> w95
            tunnel: w94 -> [w117 w251 w271 w276 w294 w303 w318 w327 w334 w371 w375 w397 w415 w420 w438 w452 w467 w475 w502 w531 w555]
            tunnel: [w117 w256 w271 w276 w294 w303 w318 w327 w334 w371 w375 w397 w415 w420 w438 w452 w467 w475 w502 w531 w555] -> w93
            tunnel: w92 -> [_ w254 _ _ _ _ _ _ _ _ _ _ _ _ _ _ _ _ _ _ _]
            event Timeout {
              n48 = event-data() -> ()  [unwired: 2 out]
              n49 = local read "offset delay"() -> (w123:dbl)
              n50 = stacked-sequence {
                seq-local: [_ w145 _] -> [_ _ w219]
                seq-local: [_ w142 _] -> [_ _ w216]
                seq-local: [_ w135 _] -> [_ _ w215]
                tunnel: w127 -> [_ w167 _]
                tunnel: [_ w166 _] -> w126
                tunnel: w125 -> [_ w165 _]
                tunnel: w124 -> [_ w162 w230]
                tunnel: "Channel tab" -> [_ w154 _]
                tunnel: w123 -> [_ w148 _]
                tunnel: w122 -> [_ w137 _]
                tunnel: [_ _ w212] -> w121
                frame #0 {
                  n51 = case shown="True" TRUE {
                    frame False {
                    }
                    frame True {
                      n52 = property class="VI"() -> (reference out=w130:refnum<vi>, "Front Panel.IsFrontmost"=w129:bool)  [unwired: 2 in, 1 out]
                      n53 = case shown="False" w129 {
                        tunnel: w130 -> [w132 _]
                        frame False {
                          n54 = property class="VI"(reference=w132, "Front Panel.IsFrontmost"=TRUE) -> ()  [unwired: 1 in, 2 out]
                        }
                        frame True {
                        }
                      }
                    }
                  }
                }
                frame #1 {
                  # "Read voltage and convery to MV. Make plot\nshowing what will be captured as RF data. Yellow\ncurser can be moved to provide addtional time shift for digitizer\ndealy."
                  # "Can View Spectrum Also"
                  n55 = expression code="1E-6*x"(w148) -> (w149:dbl)
                  n56 = case shown="\"C1\", Default" w154 {
                    tunnel: ["C1" "C2" "C3" "C4"] -> w153
                    frame "C1", Default {
                    }
                    frame "C2" {
                    }
                    frame "C3" {
                    }
                    frame "C4" {
                    }
                  }
                  n57 = call "Fetch Waveform With HZOffset.vi"("VISA resource name"=w162, "Source (0: Channel 1)"=w154, "Timeout (10000 ms)"=u32 1000, "Sparsing (0: Every point)"=1) -> ("VISA resource name out"=w150:refnum<visa-resource-name>, "Waveform Graph"=w163:waveform(dbl))  [unwired: 8 in, 2 out]
                  n58 = Unbundle By Name(w163) -> ("dt"=w147:dbl, "Y"=w144:dbl[])  [unwired: 1 out]
                  n59 = Concatenate Strings(w153, ":VDIV?" ("Write Buffer")) -> (w156:string)
                  n60 = Divide(x=w149, y=w147) -> (x/y=w142:dbl)
                  n61 = Array Size(array=w144) -> (size(s)=w145:i32)
                  n62 = Absolute Value(x=w142) -> (abs(x)=w140:dbl)
                  n63 = Reciprocal(x=w147) -> (1/x=w136:dbl)
                  n64 = call <instrlib>:"Write.vi"("Write Buffer"=w156, "VISA resource name"=w150) -> ("error out"=w157:errorcluster, "Return Count"=w158:u32, "VISA resource name out"=w159:refnum<visa-resource-name>)  [unwired: 7 in]
                  n65 = Subtract(x=w145, y=w140) -> (x-y=w143:dbl)
                  n66 = Greater Than 0?(x=w142) -> (x > 0?=w141:bool)
                  n67 = Initialize Array(0.0, w140) -> (w139:dbl[])
                  n68 = case shown="True" w141 {
                    tunnel: w144 -> [w177 w183]
                    tunnel: w143 -> [w176 w182]
                    tunnel: [w173 w178] -> w138
                    tunnel: w140 -> [_ w181]
                    tunnel: w139 -> [w174 w180]
                    frame False {
                      n69 = Array Subset(array=w177, length=w176) -> (w175:dbl[])  [unwired: 1 in]
                      n70 = Build Array (concatenate)(w174, w175) -> (w173:dbl[])
                    }
                    frame True {
                      n71 = Array Subset(array=w183, index=w181, length=w182) -> (w179:dbl[])
                      n72 = Build Array (concatenate)(w179, w180) -> (w178:dbl[])
                    }
                  }
                  n73 = call <instrlib>:"Read.vi"("error in (no error)"=w157, "Byte Count"=w158, "VISA resource name"=w159) -> ("Read Buffer"=w152:string)  [unwired: 5 in, 3 out]
                  n74 = Divide(x=10, y=w145) -> (x/y=w169:dbl)
                  n75 = Bundle By Name(cluster=w137, "Samp Rate (Hz)"=w136) -> (w135:T10)
                  n76 = expression code="1E-6*x"(w136) -> (w134:dbl)
                  n77 = Fract/Exp String To Number(string=w152) -> (number=w151:dbl)  [unwired: 3 in, 1 out]
                  n78 = case shown="True" w165 {
                    tunnel: [w193 w198] -> w164
                    tunnel: [w195 w200] -> w170
                    tunnel: w169 -> [w195 _]
                    tunnel: w167 -> [_ w203]
                    tunnel: w147 -> [_ w202]
                    tunnel: [i32[] [] w199] -> w166
                    tunnel: w138 -> [w192 w196]
                    frame False {
                      n79 = expression code="x*1000"(w192) -> (w193:dbl[])
                    }
                    frame True {
                      n80 = Transpose 2D Array(2D array=w203) -> (transposed array=w204:dbl[][])
                      n81 = for {
                        tunnel: w204 -> [w207] mode=indexing
                        tunnel: [w206] -> w197 mode=indexing
                        n82 = call-poly <vilib>:"Mean.vi"("X"=w207) -> ("mean"=w206:dbl)  [unwired: 1 out]
                      }
                      n83 = call <vilib>:"Auto Power Spectrum.vi"("dt"=w202, "Signal (V)"=w196) -> ("df"=w201:dbl, "Power Spectrum (V^2 rms)"=w199:dbl[])
                      n84 = expression code="log(x)*10"(w197) -> (w198:dbl[])
                      n85 = Multiply(x=w201, y=1e-06) -> (x*y=w200:dbl)
                    }
                  }
                  n86 = To Double Precision Float(number=w134) -> (double precision float=→"Sample Rate":dbl)
                  n87 = case shown="\"C2\"" w154 {
                    tunnel: w151 -> [w188 w189 w190 w191]
                    frame "C1", Default {
                      n88 = property on="Voltage/DIV CH1" class="DigNum (strict)"("Value"=w188) -> ()  [unwired: 2 in, 2 out]
                    }
                    frame "C2" {
                      n89 = property on="Voltage/DIV CH2" class="DigNum (strict)"("Value"=w189) -> ()  [unwired: 2 in, 2 out]
                    }
                    frame "C3" {
                      n90 = property on="Voltage/DIV CH3" class="DigNum (strict)"("Value"=w190) -> ()  [unwired: 2 in, 2 out]
                    }
                    frame "C4" {
                      n91 = property on="Voltage/DIV CH4" class="DigNum (strict)"("Value"=w191) -> ()  [unwired: 2 in, 2 out]
                    }
                  }
                  n92 = Bundle(0, w170, w164) -> (→"Waveform Graph":cluster{i32, dbl, dbl[]})  [unwired: 1 out]
                }
                frame #2 {
                  w222 = u32 15 ("Byte Count")
                  w240 = u32 1 ("Write Attribute")
                  # "Take care of data window display"
                  n93 = call <instrlib>:"Write.vi"("Write Buffer"="TDIV?", "VISA resource name"=w230) -> ("error out"=w234:errorcluster, "VISA resource name out"=w233:refnum<visa-resource-name>)  [unwired: 7 in, 1 out]
                  n94 = property on="Waveform Graph" class="WFGraph (strict)"("Active Cursor"=w240) -> ("Cursor.Cursor Position:Cursor X"=w242:dbl)  [unwired: 2 in, 2 out]
                  n95 = call <instrlib>:"Read.vi"("error in (no error)"=w234, "Byte Count"=w222, "VISA resource name"=w233) -> ("error out"=w225:errorcluster, "Read Buffer"=w231:string, "VISA resource name out"=w226:refnum<visa-resource-name>)  [unwired: 5 in, 1 out]
                  n96 = Less Than 0?(x=w242) -> (x < 0?=w241:bool)
                  n97 = Fract/Exp String To Number(string=w231) -> (number=w210:dbl)  [unwired: 3 in, 1 out]
                  n98 = case shown="True" w241 {
                    tunnel: w242 -> [w246 _]
                    tunnel: [w246 w247] -> w221
                    tunnel: w240 -> [_ w249]
                    frame False {
                    }
                    frame True {
                      w247 = 0
                      n99 = property on="Waveform Graph" class="WFGraph (strict)"("X Scale.Range:Minimum"=w247, "X Scale.Range:Maximum"=10, "Active Cursor"=w249, "Cursor.Cursor Position:Cursor X"=w247) -> ()  [unwired: 2 in, 2 out]
                    }
                  }
                  n100 = expression code="1E6*x"(w210) -> (w209:dbl)
                  n101 = call <instrlib>:"Write.vi"("error in (no error)"=w225, "Write Buffer"="TRDL?", "VISA resource name"=w226) -> ("error out"=w223:errorcluster, "VISA resource name out"=w229:refnum<visa-resource-name>)  [unwired: 6 in, 1 out]
                  n102 = property on="Time/Div" class="Ring (strict)"("Value"=w210) -> ()  [unwired: 2 in, 2 out]
                  n103 = call <instrlib>:"Read.vi"("error in (no error)"=w223, "Byte Count"=w222, "VISA resource name"=w229) -> ("Read Buffer"=w227:string)  [unwired: 5 in, 3 out]
                  n104 = Fract/Exp String To Number(string=w227) -> (number=w224:dbl)  [unwired: 3 in, 1 out]
                  n105 = expression code="-1E6*x"(w224) -> (w208:dbl)
                  n106 = Multiply(x=w209, y=w221) -> (x*y=w214:dbl)
                  n107 = property on="Delay (us)" class="DigNum (strict)"("Value"=w208) -> ()  [unwired: 2 in, 2 out]
                  n108 = Add(x=w214, y=w208) -> (x+y=w235:dbl)
                  "Total Delay (us)" <- w235
                  n109 = Divide(x=w221, y=10) -> (x/y=w218:dbl)
                  n110 = Multiply(x=w218, y=w219) -> (x*y=w217:dbl)
                  n111 = Add(x=w217, y=w216) -> (x+y=w211:dbl)
                  "read pt offset" <- w211
                  n112 = Divide(x=10, y=w219) -> (x/y=w237:dbl)
                  n113 = global read "MotionGlobals.vi" "c mm/mics"() -> (w245:sgl)
                  n114 = Multiply(x="rf points per line", y=w237) -> (x*y=w238:dbl)
                  n115 = Bundle By Name(cluster=w215, "Digitizer delay (us)"=w208, "Additional dig delay (us)"=w214, "rf points per line"="rf points per line", "LeCroyCluster.LC read pt offset"=w211) -> (w212:T10)
                  n116 = Multiply(x=w235, y=w245) -> (x*y=→"Equivalent RT delay\ndistance (mm)":dbl)
                  n117 = Add(x=w238, y=w221) -> (x+y=w239:dbl)
                  n118 = property on="Waveform Graph" class="WFGraph (strict)"("Active Cursor"=u32 0, "Cursor.Cursor Position:Cursor X"=w239) -> ()  [unwired: 2 in, 2 out]
                }
              }
            }
            event "T/R Channel": Value Change {
              n119 = event-data() -> ("NewVal"=w253:u32)  [unwired: 2 out]
              n120 = case shown="\"No Switch\", Default" w254 {
                tunnel: w253 -> [w257 w261]
                tunnel: w252 -> [_ w260]
                tunnel: w250 -> [_ w259]
                frame "Cytex" {
                  n121 = call "Cytex.vi"("Xmit Ring"=w257) -> ()  [unwired: 2 in, 3 out]
                }
                frame "No Switch", Default {
                  # "Turn off transmits except for selected"
                  n122 = Unbundle By Name(w259) -> ("Dig Config"=w258:T12)
                  n123 = case shown="\"5-CH Pulser New\"" w258 {
                    tunnel: w261 -> [_ w266]
                    tunnel: w260 -> [_ w262]
                    frame "Single channel", Default {
                    }
                    frame "5-CH Pulser New" {
                      n124 = Decrement(x=w266) -> (x-1=w265:u32)
                      n125 = expression code="1E6/x"(w262) -> (w263:dbl)
                      n126 = Replace Array Subset(array=i32[] [-1, -1, -1, -1, -1], new element=0, index=w265) -> (w268:i32[])
                      n127 = Build Array(w268) -> (w267:i32[][])
                      n128 = global read "PulserGlobals.vi" "Daxsonics VISA"() -> (w270:refnum<visa-resource-name>)
                      n129 = call "DelayTableLoad.vi"("PRI (ns)"=w263, "Delay Table (ns)"=w267, "VISA Refnum in"=w270) -> ()  [unwired: 9 in]
                    }
                  }
                }
              }
              n130 = Bundle By Name(cluster=w251, "Switch T/R"=w253) -> (w256:T2)
            }
            event "Channel tab": Value Change {
              w272 = u8 1 ("Y Scale.Scale Fit")
              n131 = event-data() -> ()  [unwired: 2 out]
              n132 = property on="Waveform Graph" class="WFGraph (strict)"("XScale.ScaleFit"=w272, "YScale.ScaleFit"=w272) -> ()  [unwired: 2 in, 2 out]
            }
            event "Voltage/DIV CH1", "Voltage/DIV CH3", "Voltage/DIV CH4", "Voltage/DIV CH2": Value Change {
              n133 = event-data() -> ()  [unwired: 7 out]
              n134 = property on="Channel tab" class="TabCtl (strict)"() -> ("Value"=w280:enum32{"C1", "C2", "C3", "C4"})  [unwired: 2 in, 2 out]
              n135 = case shown="\"C4\"" w280 {
                tunnel: ["C1:" "C2:" "C3:" "C4:"] -> w279
                tunnel: ["Voltage/DIV CH1" "Voltage/DIV CH2" "Voltage/DIV CH3" "Voltage/DIV CH4"] -> w278
                frame "C1", Default {
                }
                frame "C2" {
                }
                frame "C3" {
                }
                frame "C4" {
                }
              }
              n136 = Format Into String(format string="%sVDIV %.;%g;", w279, w278) -> (resulting string=w277:string)  [unwired: 2 in, 1 out]
              n137 = call <instrlib>:"Write.vi"("Write Buffer"=w277, "VISA resource name"=w282) -> ()  [unwired: 7 in, 3 out]
            }
            event "Delay (us)": Value Change {
              n138 = event-data() -> ()  [unwired: 7 out]
              n139 = expression code="-x*(1e-6)"("Delay (us)") -> (w297:dbl)
              n140 = Format Into String(format string="TRDL %e", w297) -> (resulting string=w296:string)  [unwired: 2 in, 1 out]
              n141 = call <instrlib>:"Write.vi"("Write Buffer"=w296, "VISA resource name"=w295) -> ()  [unwired: 7 in, 3 out]
            }
            event "Time/Div": Value Change {
              # "TIMEBASE COMMAND"
              n142 = event-data() -> ("NewVal"=w305:dbl)  [unwired: 2 out]
              n143 = Unbundle By Name(w310) -> ("Additional dig delay (us)"=w311:dbl)
              n144 = expression code="x*1e6"(w305) -> (w304:dbl)
              n145 = Divide(x=w311, y=w304) -> (x/y=w307:dbl)
              n146 = In Range and Coerce(upper limit=9.9, x=w307, lower limit=0.0) -> (coerced(x)=w306:dbl)  [unwired: 1 out]
              n147 = Format Into String(format string="TDIV %.;%g;", w305) -> (resulting string=w314:string)  [unwired: 2 in, 1 out]
              n148 = property on="Waveform Graph" class="WFGraph (strict)"("Active Cursor"=u32 1, "Cursor.Cursor X"=w306) -> ()  [unwired: 2 in, 2 out]
              n149 = call <instrlib>:"Write.vi"("Write Buffer"=w314, "VISA resource name"=w313) -> ()  [unwired: 7 in, 3 out]
            }
            event "Delay Corr?": Value Change {
              n150 = event-data() -> ()  [unwired: 4 out]
              n151 = call "PulserSettingsSwitch.vi"("Pulser"=w324, "Digitizer Settings in"=w322, "Offset delay (us)"="offset delay", "Delay Corr?"="Delay Corr?") -> ("Digitizer Settings out"=w320:T10)  [unwired: 9 in, 2 out]
              n152 = Unbundle By Name(w320) -> ("Digitizer delay (us)"=w319:dbl)
              n153 = property on="offset delay" class="DigNum (strict)"("Value"=w319) -> ()  [unwired: 2 in, 2 out]
            }
            event "Set Pulser": Value Change {
              # "set up Panametrics if option is selected"
              n154 = event-data() -> ()  [unwired: 2 out]
              n155 = call "SetAllPulsersGUI.vi"("Init Tabor?"=FALSE ("Init?"), "Tabor handle in"=w331, "Pulser"=w329) -> ()  [unwired: 9 in]
            }
            event "Load Lecroy Setup": Value Change {
              w338 = u16 3 items=["Channel 1", "Channel 2", "Channel 3", "Channel 4", "External", "Line", "Ext", "Ext10"] ("Trigger Source (0: Channel 1)")
              w348 = u16 2 items=["A1M", "D1M", "D50", "Ground", "DC", "AC"] ("Vertical Coupling (0: A1M)")
              w349 = u16 0 items=["Channel 1", "Channel 2", "Channel 3", "Channel 4"] ("Channel (0: Channel 1)")
              n156 = event-data() -> ()  [unwired: 7 out]
              n157 = case shown="\"500 MHz New\"" "Lecroy Setup" {
                tunnel: [0.066 ("Vertical Range (10.0 V)") 0.085 ("Vertical Range (10.0 V)") 0.068 ("Vertical Range (10.0 V)") 0.176 ("Vertical Range (10.0 V)") 0.136 ("Vertical Range (10.0 V)") 0.0365 ("Vertical Range (10.0 V)")] -> w347
                tunnel: [2e-08 ("Timebase (0.0005 s)") 2e-08 ("Timebase (0.0005 s)") 5e-09 ("Timebase (0.0005 s)") 5e-09 ("Timebase (0.0005 s)") 5e-09 ("Timebase (0.0005 s)") 5e-07 ("Timebase (0.0005 s)")] -> w343
                tunnel: [-1.6744e-06 ("Position (0.0 s)") -1.5136e-06 ("Position (0.0 s)") 0.0 ("Position (0.0 s)") -5.545e-07 ("Position (0.0 s)") -5.488e-07 ("Position (0.0 s)") 9e-08 ("Position (0.0 s)")] -> w342
                frame "250 MHz Focus" {
                }
                frame "Opti 250" {
                }
                frame "500 MHz" {
                }
                frame "500 MHz Focus" {
                }
                frame "500 MHz New" {
                }
                frame "250 MHz" {
                }
              }
              n158 = expression code="x*8"(w347) -> (w337:dbl)
              n159 = call <instrlib>:"Configure Channel.vi"("VISA resource name"=w336, "Enable Channel (T:On)"=TRUE, "Channel (0: Channel 1)"=w349, "Vertical Coupling (0: A1M)"=w348, "Vertical Range (10.0 V)"=w337) -> ("VISA resource name out"=w344:refnum<visa-resource-name>, "error out"=w345:errorcluster)  [unwired: 9 in]
              n160 = call <instrlib>:"Configure Timebase.vi"("error in (no error)"=w345, "Position (0.0 s)"=w342, "Timebase (0.0005 s)"=w343, "VISA resource name"=w344) -> ("error out"=w340:errorcluster, "VISA resource name out"=w341:refnum<visa-resource-name>)  [unwired: 6 in]
              n161 = call-poly <instrlib>:"Configure Trigger.vi"("VISA resource name"=w341, "Trigger Source (0: Channel 1)"=w338, "Trigger Level (0.0 V)"=3.0, "error in (no error)"=w340) -> ()  [unwired: 10 in, 2 out]
            }
            event "Custom Waveform": Value Change {
              n162 = event-data() -> ()  [unwired: 3 out]
              n163 = call "Chirp.vi"() -> ()  [unwired: 6 in, 1 out]
            }
            event "Man Cont": Value Change {
              n164 = event-data() -> ()  [unwired: 2 out]
              n165 = Unbundle By Name(w379) -> ("Motion System"=w378:T7)
              n166 = case shown="\"NI 735x\", Default" w378 {
                tunnel: w379 -> [w382 w384 w390 w393 w395]
                tunnel: [w382 w383 w389 w392 w395] -> w377
                frame "MM3000" {
                }
                frame "NI 735x", Default {
                  n167 = disable-structure shown="Enabled" {
                    disable-tunnel: w384 -> [w386 w388]
                    disable-tunnel: [w385 w388] -> w383
                    frame Disabled {
                      n168 = call "NI_controller.VI"("Motion Settings"=w386, "Initialize"=FALSE) -> ("Motion Settings Out"=w385:T6)  [unwired: 3 in, 1 out]
                    }
                    frame Enabled {
                    }
                  }
                }
                frame "Galil" {
                  n169 = call "GL_controller.VI"("Motion Settings"=w390, "Initialize"=FALSE) -> ("Motion Settings Out"=w389:T6)  [unwired: 3 in, 1 out]
                }
                frame "Newport ESP" {
                  n170 = call "ESPControl.vi"("Motion Settings"=w393, "# Axis"=u16 2) -> ("Motion Settings Out"=w392:T6)  [unwired: 3 in, 1 out]
                }
                frame "No Motion Card" {
                }
              }
              n171 = local read "Axis"() -> (w381:enum32{"Axis 1", "Axis 2", "Axis 3", "Axis 4"})
              n172 = property on="Axis" class="RadioBtnsControl (strict)"("Val(Sgnl)"=w381) -> ()  [unwired: 2 in, 2 out]
            }
            event Key Down {
              n173 = event-data() -> ("VKey"=w407:T22, "Char"=w408:i16, "PlatMods"=w412:T23)  [unwired: 1 out]
              n174 = property on="prf (kHz)" class="DigNum (strict)"() -> ("Key Focus"=w398:bool)  [unwired: 2 in, 2 out]
              n175 = property on="Inc Step\nSize (mm)" class="DigNum (strict)"() -> ("Key Focus"=w399:bool)  [unwired: 2 in, 2 out]
              n176 = property on="Gate duration (mics)" class="DigNum (strict)"() -> ("Key Focus"=w404:bool)  [unwired: 2 in, 2 out]
              n177 = property on="rf points per line" class="DigNum (strict)"() -> ("Key Focus"=w403:bool)  [unwired: 2 in, 2 out]
              n178 = property on="Delay (us)" class="DigNum (strict)"() -> ("Key Focus"=w402:bool)  [unwired: 2 in, 2 out]
              n179 = property on="Position (mm) (Abs)" class="DigNum (strict)"() -> ("Key Focus"=w401:bool)  [unwired: 2 in, 2 out]
              n180 = Compound Arithmetic op=OR(w398, w399, w404, w403, w402, w401) -> (w400:bool)
              n181 = control-ref of="Axis"() -> (w411:refnum<vi>)
              n182 = control-ref of="Waveform Graph"() -> (w410:refnum<vi>)
              n183 = control-ref of="Position (mm) (Abs)"() -> (w409:refnum<vi>)
              n184 = call "KeyboardNudge.vi"("WaveformGraph Refnum"=w410, "Axis Tune Refnum"=w411, "Char"=w408, "Position (mm) Refnum"=w409, "Ignore Key Down"=w400, "VKey"=w407, "PlatMods"=w412, "Inc. Step Size (mm)"=w406, "Motion Settings"=w396) -> ("Quit"=w405:bool)  [unwired: 9 in, 1 out]
            }
            event "prf (kHz)": Value Change {
              n185 = event-data() -> ()  [unwired: 7 out]
              n186 = global write "PulserGlobals.vi" "prf (kHz)"("prf (kHz)") -> ()
            }
            event "Save trace?": Value Change {
              n187 = event-data() -> ()  [unwired: 2 out]
              n188 = local read "Waveform Graph"() -> (w426:cluster{i32, dbl, dbl[]})
              n189 = Unbundle(w426) -> (w434:dbl, w433:dbl[])  [unwired: 1 out]
              n190 = local read "Time/Div"() -> (w425:dbl)
              n191 = for {
                tunnel: w434 -> [w436]
                tunnel: w433 -> [_] mode=indexing
                tunnel: [w435] -> w431 mode=indexing
                i -> [w437]
                n192 = Multiply(x=w436, y=w437) -> (x*y=w435:dbl)
              }
              n193 = Select(t=1, s=w427, f=w425) -> (s? t:f=w428:dbl)
              n194 = Multiply(x=w431, y=w428) -> (x*y=w430:dbl[])
              n195 = Build Array(w430, w433) -> (w432:dbl[][])
              n196 = Transpose 2D Array(2D array=w432) -> (transposed array=w422:dbl[][])
              n197 = call-poly <vilib>:"Write Delimited Spreadsheet.vi"("2D data"=w422) -> ()  [unwired: 13 in, 2 out]
            }
            event "Therapy Burst Set Up.Divide prf by", "Therapy Burst Set Up.Therapy Delay (ms)", "Gate duration (mics)": Value Change {
              n198 = event-data() -> ()  [unwired: 2 out]
              n199 = Unbundle("Therapy Burst Set Up") -> ("Therapy Set Up"=w448:T24, "Divide prf by"=w449:i32, "Therapy Delay (ms)"=w450:dbl, "Counter On (T)"=w442:bool)
              n200 = Unbundle By Name(w448) -> ("Cycles"=w446:sgl)
              n201 = Multiply(x="Gate duration (mics)", y=1e-06) -> (x*y=w444:dbl)
              n202 = Multiply(x=w441, y=w446) -> (x*y=→"Lines in burst":dbl)
              n203 = call "ExtPRFCount.vi"("Therapy Delay (ms)"=w450, "Start Counter?"=w442, "Divide prf by"=w449, "pulse width (s or cycles)"=w444) -> ()  [unwired: 12 out]
            }
            event "Therapy Burst Set Up.Therapy Set Up": Value Change {
              # "Set up burst parameters"
              # "Pause Therapy if needed."
              n204 = event-data() -> ("NewVal"=w458:T24)  [unwired: 1 out]
              n205 = global read "MotionGlobals.vi" "33250(T)/33120(F)"() -> (w455:bool)
              n206 = case shown="1" "Func Gen" {
                tunnel: w458 -> [w464 w466]
                tunnel: "cycles (f), time(t)" -> [w463 _]
                tunnel: w460 -> [_ w465]
                tunnel: w455 -> [w461 _]
                frame 0, Default {
                  n207 = call "TherapyBurst.vi"("Input Cluster"=w464, "VISA session in"="Therapy VISA session", "33250(T)/33120(F)"=w461, "Trigger (F) Gate(T)"=w463) -> ()  [unwired: 1 in, 4 out]
                }
                frame 1 {
                  n208 = call "TaborBurst.vi"("Input Cluster"=w466, "instrument in"=w465) -> ()  [unwired: 1 in, 6 out]
                }
              }
            }
            event "Therapy Burst Set Up.Counter On (T)": Value Change {
              n209 = event-data() -> ("NewVal"=w472:bool)  [unwired: 1 out]
              n210 = global read "MotionGlobals.vi" "DAQmx Task 1"() -> (w471:refnum<k21>)
              n211 = case shown="True" w472 {
                tunnel: w471 -> [w473 w474]
                frame False {
                  n212 = call <vilib>:"DAQmx Stop Task.vi"("task/channels in"=w473) -> ()  [unwired: 1 in, 14 out]
                }
                frame True {
                  n213 = call <vilib>:"DAQmx Start Task.vi"("task/channels in"=w474) -> ()  [unwired: 1 in, 14 out]
                }
              }
            }
            event "ExitSendCmd": Value Change {
              n214 = event-data() -> ()  [unwired: 2 out]
              n215 = property on="Waveform Graph" class="WFGraph (strict)"("Active Cursor"=u32 0) -> ("Cursor.Cursor X"=w485:dbl)  [unwired: 2 in, 2 out]
              n216 = Less Or Equal?(x=w485, y=10) -> (x <= y?=w482:bool)
              n217 = case shown="False" w482 {
                tunnel: [w488 TRUE] -> w481
                frame False {
                  n218 = Two Button Dialog(message="WARNING! Red line goes beyond right side of window. Adjust time base so more points are available or adjust window location. ", 1:"Override" ("F button name (\"Cancel\")")) -> (T button?=w489:bool)  [unwired: 1 in]
                  n219 = Not(x=w489) -> (.not. x?=w488:bool)
                }
                frame True {
                }
              }
              n220 = property on="ExitSendCmd" class="Bool (strict)"("Value"=FALSE ("ExitSendCmd")) -> ()  [unwired: 2 in, 2 out]
              n221 = And(x="ExitSendCmd", y=w481) -> (x .and. y?=w476:bool)
            }
            event "Position (mm) (Abs)": Value Change {
              n222 = event-data() -> ()  [unwired: 2 out]
              n223 = Unbundle By Name(w492) -> ("Reverse Z axis?"=w496:bool, "Steps per mm"=w501:i32[])
              n224 = local read "Axis"() -> (w500:enum32{"Axis 1", "Axis 2", "Axis 3", "Axis 4"})
              n225 = Index Array(array=w501, index=w500) -> (element=w499:i32)
              n226 = To Byte Integer(number=w500) -> (8bit integer=w494:i8)
              n227 = Multiply(x="Position (mm) (Abs)", y=w499) -> (x*y=w497:dbl)
              n228 = case shown="\"Axis 3\"" w500 {
                tunnel: w497 -> [w505 w508]
                tunnel: [w505 w506] -> w495
                tunnel: w496 -> [_ w507]
                frame "Axis 1", Default {
                }
                frame "Axis 3" {
                  n229 = Negate(x=w508) -> (-x=w509:dbl)
                  n230 = Select(t=w509, s=w507, f=w508) -> (s? t:f=w506:dbl)
                }
              }
              n231 = Unbundle By Name(w492) -> ("Motion System"=w493:T7)
              n232 = case shown="\"NI 735x\", Default" w493 {
                tunnel: w492 -> [_ w510 w517]
                tunnel: w495 -> [_ w512 w516]
                tunnel: w494 -> [_ w511 w515]
                frame "MM3000", "Newport ESP", "No Motion Card" {
                }
                frame "Galil" {
                  n233 = Unbundle By Name(w510) -> ("GL Ref Out"=w514:refnum<k7>)
                  n234 = call "GL Set Operation Mode.vi"("position cts (abs/rel)"=w512, "Start Now?"=TRUE, "Axis"=w511, "Galil.IGalil"=w514) -> ()  [unwired: 5 in, 3 out]
                }
                frame "NI 735x", Default {
                  n235 = disable-structure shown="Disabled" {
                    disable-tunnel: w517 -> [w522 _]
                    disable-tunnel: w516 -> [w520 _]
                    disable-tunnel: w515 -> [w519 _]
                    frame Disabled {
                      n236 = Unbundle By Name(w522) -> ("Motion Bd ID"=w521:u8)
                      n237 = Increment(x=w519) -> (x+1=w518:i8)
                      n238 = call <vilib>:"Set Operation Mode.flx"("Axis or Vector Space"=w518, "Board ID"=w521) -> ("error out"=w528:errorcluster, "Resource Output"=w526:T25, "Bd ID Out"=w527:T26)  [unwired: 4 in]
                      n239 = call <vilib>:"Load Target Position.flx"("Target Position (0)"=w520, "error in (no error)"=w528, "Axis"=w526, "Board ID"=w527) -> ("error out"=w524:errorcluster, "Resource Output"=w523:T25, "Bd ID Out"=w525:T26)  [unwired: 3 in]
                      n240 = call-poly <vilib>:"Start Motion.flx"("error in (no error)"=w524, "Axis or Vector Space"=w523, "Board ID"=w525) -> ()  [unwired: 3 in, 3 out]
                    }
                    frame Enabled {
                    }
                  }
                }
              }
            }
            event "Stop Motor": Value Change {
              n241 = event-data() -> ()  [unwired: 2 out]
              n242 = Unbundle By Name(w530) -> ("Motion System"=w529:T7)
              n243 = case shown="\"NI 735x\"" w529 {
                tunnel: w530 -> [w535 w538 w545]
                tunnel: [w535 w536 w544] -> w533
                frame "MM3000", Default {
                }
                frame "Galil" {
                  n244 = Unbundle By Name(w538) -> ("GL Ref Out"=w540:refnum<k7>)
                  n245 = call "GL Command Set.vi"("Command"=Command_Menu."Abort Motion", "Galil.IGalil"=w540) -> ("error out"=w539:errorcluster)  [unwired: 5 in, 4 out]
                  n246 = call "FindLocation.vi"("Motion Settings"=w538, "error in (no error)"=w539) -> ("Motion Settings Out"=w536:T6, "location (mm)"=w543:dbl[])  [unwired: 1 in, 2 out]
                  n247 = local read "Axis"() -> (w541:enum32{"Axis 1", "Axis 2", "Axis 3", "Axis 4"})
                  n248 = Index Array(array=w543, index=w541) -> (element=w537:dbl)
                  n249 = local write "Position (mm) (Abs)"(w537) -> ()
                }
                frame "NI 735x" {
                  n250 = disable-structure shown="Disabled" {
                    disable-tunnel: w545 -> [w547 _]
                    disable-tunnel: [w546 _] -> w544
                    frame Disabled {
                      n251 = Unbundle By Name(w547) -> ("Motion Bd ID"=w548:u8)
                      n252 = local read "Axis"() -> (w552:enum32{"Axis 1", "Axis 2", "Axis 3", "Axis 4"})
                      n253 = Increment(x=w552) -> (x+1=w549:enum32{"Axis 1", "Axis 2", "Axis 3", "Axis 4"})
                      n254 = call-poly <vilib>:"Stop Motion.flx"("Stop Type (Decel)"=enum16{"Decelerate", "Halt", "Kill"}."Halt", "Axis or Vector Space"=w549, "Board ID"=w548) -> ("error out"=w551:errorcluster)  [unwired: 4 in, 2 out]
                      n255 = call "FindLocation.vi"("Motion Settings"=w547, "error in (no error)"=w551) -> ("Motion Settings Out"=w546:T6, "location (mm)"=w553:dbl[])  [unwired: 1 in, 2 out]
                      n256 = Index Array(array=w553, index=w552) -> (element=w554:dbl)
                      n257 = local write "Position (mm) (Abs)"(w554) -> ()
                    }
                    frame Enabled {
                    }
                  }
                }
              }
            }
            event "Axis": Value Change {
              n258 = event-data() -> ()  [unwired: 2 out]
              n259 = Unbundle By Name(w559) -> ("Motion System"=w558:T7)
              n260 = case shown="\"NI 735x\", Default" w558 {
                tunnel: w559 -> [w562 w566]
                tunnel: [w561 w566] -> w557
                frame "NI 735x", Default {
                  n261 = call "FindLocation.vi"("Motion Settings"=w562) -> ("Motion Settings Out"=w561:T6, "location (mm)"=w565:dbl[])  [unwired: 2 in, 2 out]
                  n262 = Index Array(array=w565, index="Axis") -> (element=w564:dbl)
                  n263 = local write "Position (mm) (Abs)"(w564) -> ()
                }
                frame "MM3000", "Newport ESP", "No Motion Card" {
                }
              }
            }
          }
          n264 = Build Array (concatenate)(w116, w109) -> (w115:dbl[][])
          n265 = Array Subset(array=w115, length (row)=20) -> (w114:dbl[][])  [unwired: 3 in]
        }
      }
      frame #2 {
        # "update with last location"
        # "turn off prf"
        # "Stop counter afte therapy burst or EKG modes"
        n266 = Not Equal To 0?(x=w574) -> (x != 0?=w571:bool)
        n267 = Compound Arithmetic op=OR(w570, w569, w572, w571) -> (w573:bool)
        n268 = case shown="True" w573 {
          frame False {
          }
          frame True {
            n269 = global read "MotionGlobals.vi" "DAQmx Task 1"() -> (w576:refnum<k21>)
            n270 = call <vilib>:"DAQmx Stop Task.vi"("task/channels in"=w576) -> ()  [unwired: 1 in, 14 out]
          }
        }
        n271 = call "PRF_Off.vi"("Location"=w575, "Motion Settings In"=w567) -> ()  [unwired: 9 in, 1 out]
        n272 = call <instrlib>:"ww128x Close.vi"("instrument handle"=w568) -> ()  [unwired: 10 in, 1 out]
      }
    }
  }
  "Digitizer Settings Out" <- w8
  "Motion Settings Out" <- w6
  "Ann Array Params out" <- w2
